vi "fruit.add.vi"(8 "error in (no error)":errorcluster, 10 "Fruit.lvclass":refnum<class "Fruit.lvclass">, 11 "Game Board in":refnum<class "Game Board.lvclass">) -> (0 "error out":errorcluster, 3 "Game Board out":refnum<class "Game Board.lvclass">)   [LabVIEW 2020, in "Game Board.lvclass"]
uses:
  Game Board.lvclass
  Fruit/Fruit.lvclass
  Game Board.lvclass/Game Board.ctl
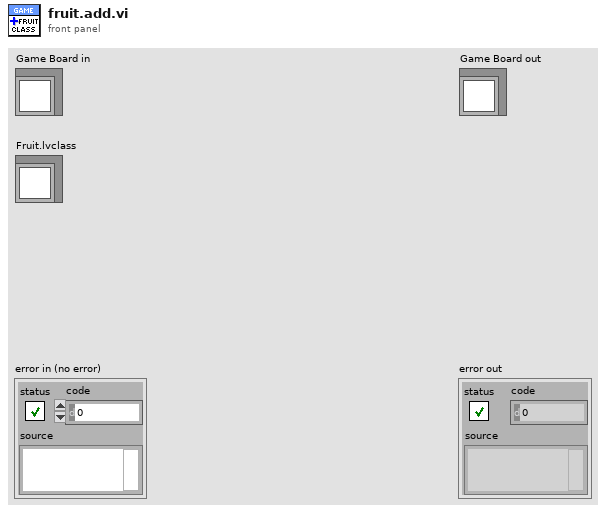
[diagram p1: front panel]
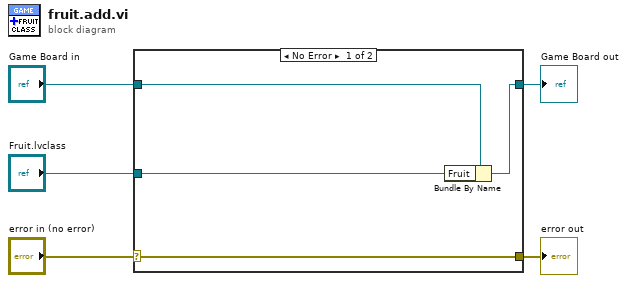
[diagram p0: block diagram]
diagram:
  n1 = case shown="No Error" "error in (no error)" {
    selector: "error in (no error)" -> [w9 w10]
    tunnel: [w9 w10] -> w4
    tunnel: [w7 w11] -> w2
    tunnel: "Game Board in" -> [w8 w11]
    tunnel: "Fruit.lvclass" -> [w6 _]
    frame No Error {
      n2 = Bundle By Name(cluster=w8, "Fruit"=w6) -> (w7:refnum<class "Game Board.lvclass">)
    }
    frame Error {
    }
  }
  "error out" <- w4
  "Game Board out" <- w2
